vi "PI release semaphore.vi"(0 "System no.":i32=1 min=1 step=1, 2 "timed out":bool, 3 "semaphore":T1, 5 "error in":errorcluster) -> (19 "error out":errorcluster)   [LabVIEW 2020]
doc: "This VI releases the semaphore that was defined in Global1.vi for the specified system."
panel:
  # "This vi releases the semaphore that was defined in Global1.vi for the specified system."
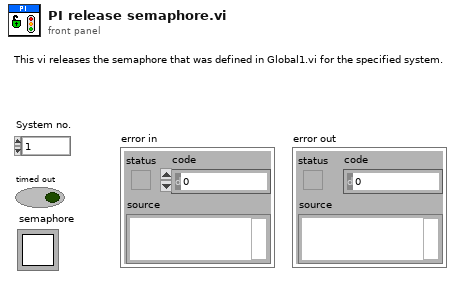
[diagram p1: front panel]
types:
  T1 = typedef "Semaphore RefNum" = refnum<k1>
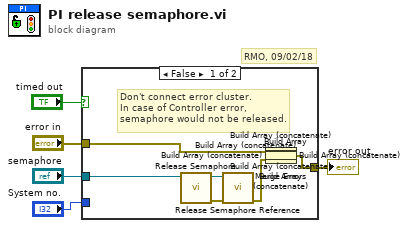
[diagram p0: block diagram]
diagram:
  # "RMO, 09/02/18"
  n1 = case shown="False" "timed out" {
    tunnel: [w17 w19] -> w3
    tunnel: "error in" -> [w18 w19]
    tunnel: "System no." -> [_ _]
    tunnel: "semaphore" -> [w16 _]
    frame False {
      # "Don't connect error cluster.\nIn case of Controller error,\nsemaphore would not be released."
      n2 = call <vilib>:"Release Semaphore.vi"("semaphore"=w16) -> ("error out"=w15:errorcluster, "semaphore out"=w13:T1)  [unwired: 1 in, 4 out]
      n3 = call <vilib>:"Release Semaphore Reference.vi"("error in (no error)"=w15, "semaphore"=w13) -> ("error out"=w14:errorcluster)  [unwired: 9 out]
      n4 = Build Array(w18, w14) -> (w12:errorcluster[])
      n5 = Build Array (concatenate)(w12) -> (w11:errorcluster[])
      n6 = Build Array (concatenate)(w11) -> (w10:errorcluster[])
      n7 = Build Array (concatenate)(w10) -> (w9:errorcluster[])
      n8 = Build Array (concatenate)(w9) -> (w8:errorcluster[])
      n9 = Build Array (concatenate)(w8) -> (w7:errorcluster[])
      n10 = Build Array (concatenate)(w7) -> (w6:errorcluster[])
      n11 = Merge Errors(w6) -> (w17:errorcluster)
    }
    frame True {
      # "timed out"
    }
  }
  "error out" <- w3
